vi "Init Events.vi"(8 "error in (no error)":errorcluster, 11 "ControlArray in":refnum<class "ControlArray.lvclass">) -> (0 "error out":errorcluster, 3 "ControlArray out":refnum<class "ControlArray.lvclass">)   [LabVIEW 2020, in "Control Array.lvlib" / "ControlArray.lvclass"]
uses:
  ControlArray.lvclass
  Element Changed Event Data.ctl
  ControlArray.lvclass/ControlArray.ctl
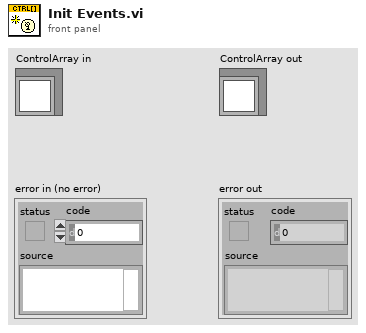
[diagram p1: front panel]
types:
  T1 = typedef "Control Array.lvlib/ControlArray.lvclass/Element Changed Event Data.ctl" = cluster{"Value":variant, "Index":i32, "Ctl Ref":refnum<vi>}
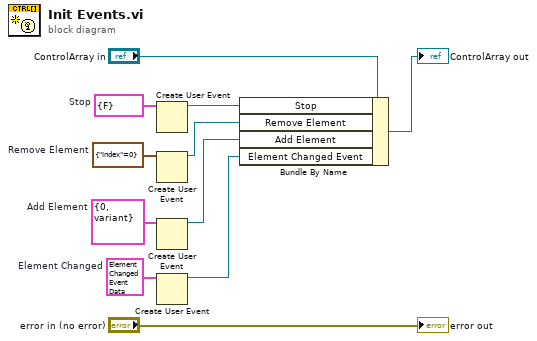
[diagram p0: block diagram]
diagram:
  w7 = cluster{"Index":i32, "Value":variant} {"Index"=0, "Value"=variant}  # Add Element
  w8 = cluster{"Index":i32} {"Index"=0}  # Remove Element
  w9 = cluster{"Stop":bool} {"Stop"=FALSE}  # Stop
  w10 = T1 {"Value"=variant, "Index"=0, "Ctl Ref"=refnum}  # Element Changed
  n1 = Create User Event(user event datatype=w9) -> (user event=w5:refnum<user-event>)  [unwired: 1 in, 1 out]
  n2 = Create User Event(user event datatype=w8) -> (user event=w4:refnum<user-event>)  [unwired: 1 in, 1 out]
  n3 = Create User Event(user event datatype=w7) -> (user event=w3:refnum<user-event>)  [unwired: 1 in, 1 out]
  n4 = Create User Event(user event datatype=w10) -> (user event=w2:refnum<user-event>)  [unwired: 1 in, 1 out]
  n5 = Bundle By Name(cluster="ControlArray in", "Stop"=w5, "Remove Element"=w4, "Add Element"=w3, "Element Changed Event"=w2) -> (→"ControlArray out":refnum<class "ControlArray.lvclass">)
  "error out" <- "error in (no error)"
